vi "jacks_out_v3.vi"(0 "J4 DOWN":bool, 1 "J4 UP":bool, 2 "J3 DOWN":bool, 3 "J3 UP":bool, 4 "J2 DOWN":bool, 5 "J2 UP":bool, 6 "J1 DOWN":bool, 7 "J1 UP":bool) -> ()   [LabVIEW 2019]
uses:
  <vilib>/myRIO/Instrument Drivers/Onboard IO/UART/typedef/VISA Configuration.ctl
  <vilib>/Instr/_visa.llb/VISA Configure Serial Port (Instr).vi
  <vilib>/myRIO/Instrument Drivers/Onboard IO/UART/UART.lvlib
panel:
  out "resulting string":string
  out "Characters Read":string
  out "Character Count":u32
  in  "error in (no error)":errorcluster
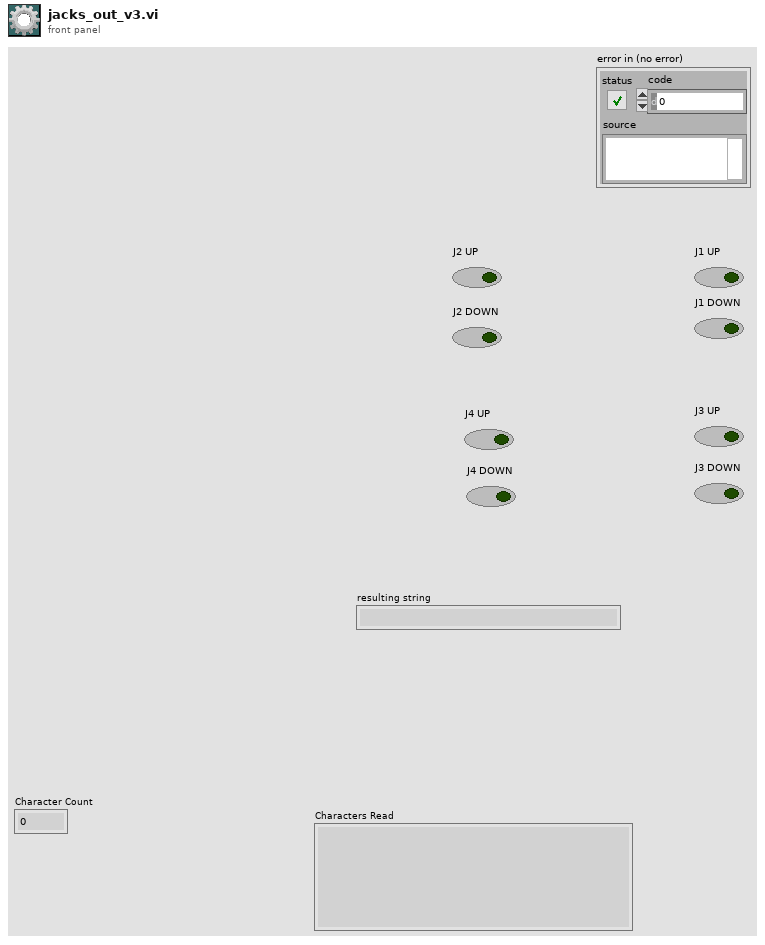
[diagram p1: front panel]
types:
  T1 = typedef "UART.lvlib/VISA Configuration.ctl" = cluster{"baud rate (9600)":u32, "data bits (8)":u16, "parity (0:none)":enum16{"None", "Odd", "Even", "Mark", "Space"}, "stop bits (10: 1 bit)":u16, "flow control (0:none)":u16, "termination char\n(0xA = '\\n' = LF) ":u8, "Enable Termination\nChar (T)":bool, "timeout (10sec)":u32}
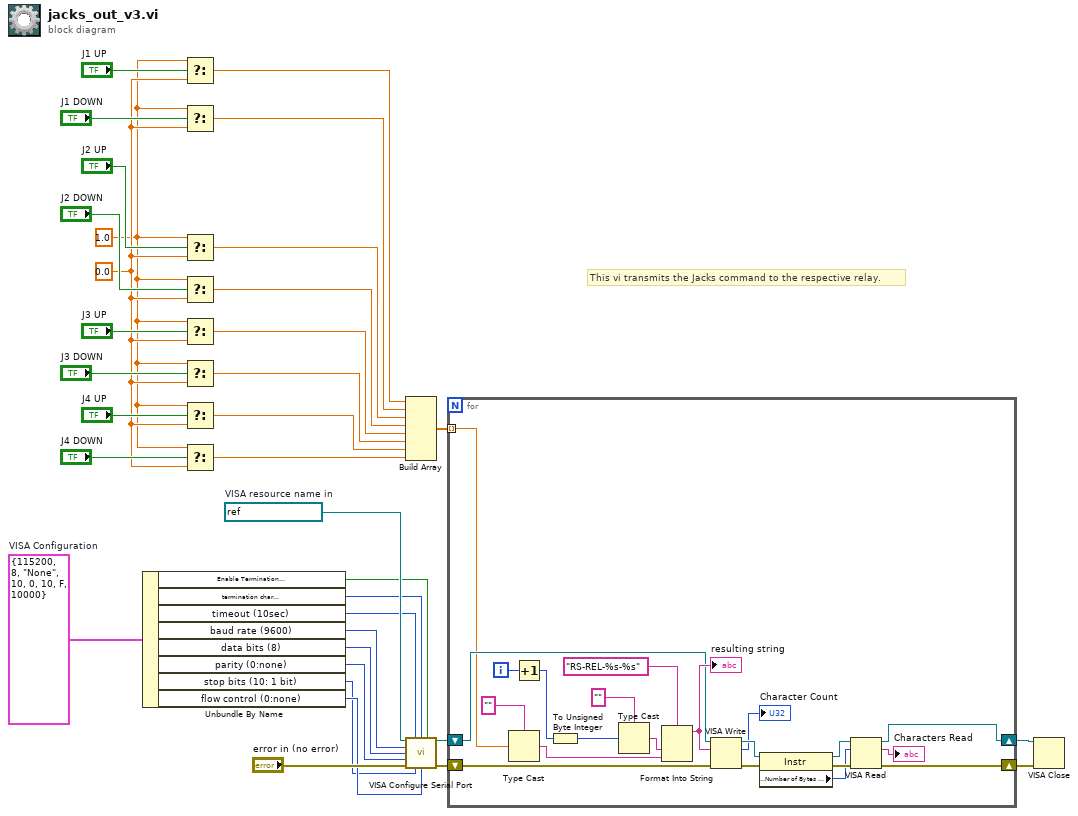
[diagram p0: block diagram]
diagram:
  w14 = 0.0 ("f")
  w13 = 1.0 ("t")
  w33 = T1 {"baud rate (9600)"=115200, "data bits (8)"=8, "parity (0:none)"=enum."None", "stop bits (10: 1 bit)"=10, "flow control (0:none)"=0, "termination char\n(0xA = '\\n' = LF) "=10, "Enable Termination\nChar (T)"=FALSE, "timeout (10sec)"=10000}  # VISA Configuration
  w34 = refnum<visa-resource-name> "ASRL2::INSTR"  # VISA resource name in
  # "This vi transmits the Jacks command to the respective relay."
  n1 = Unbundle By Name(w33) -> ("Enable Termination\nChar (T)"=w31:bool, "termination char\n(0xA = '\\n' = LF)"=w30:u8, "timeout (10sec)"=w29:u32, "baud rate (9600)"=w24:u32, "data bits (8)"=w25:u16, "parity (0:none)"=w26:enum16{"None", "Odd", "Even", "Mark", "Space"}, "stop bits (10: 1 bit)"=w27:u16, "flow control (0:none)"=w28:u16)
  n2 = Select(t=w13, s="J1 UP", f=w14) -> (s? t:f=w12:dbl)
  n3 = Select(t=w13, s="J1 DOWN", f=w14) -> (s? t:f=w11:dbl)
  n4 = Select(t=w13, s="J2 UP", f=w14) -> (s? t:f=w10:dbl)
  n5 = Select(t=w13, s="J2 DOWN", f=w14) -> (s? t:f=w9:dbl)
  n6 = Select(t=w13, s="J3 UP", f=w14) -> (s? t:f=w8:dbl)
  n7 = Select(t=w13, s="J3 DOWN", f=w14) -> (s? t:f=w7:dbl)
  n8 = Select(t=w13, s="J4 UP", f=w14) -> (s? t:f=w6:dbl)
  n9 = Select(t=w13, s="J4 DOWN", f=w14) -> (s? t:f=w5:dbl)
  n10 = Build Array(w12, w11, w10, w9, w8, w7, w6, w5) -> (w4:dbl[])
  n11 = call-poly "VISA Configure Serial Port"("VISA resource name"=w34, "timeout (10sec)"=w29, "termination char\n(0xA = '\\n' = LF)"=w30, "Enable Termination\nChar (T)"=w31, "baud rate (9600)"=w24, "data bits (8)"=w25, "parity (0:none)"=w26, "error in (no error)"="error in (no error)", "stop bits (10: 1 bit)"=w27, "flow control (0:none)"=w28) -> ("VISA resource name out"=w15:refnum<visa-resource-name>, "error out"=w1:errorcluster)  [unwired: 4 in]
  n12 = for {
    shift-right: [w37] -> w3
    shift-left: w15 -> [w41]
    tunnel: w4 -> [w39] mode=indexing
    shift-right: [w36] -> w2
    shift-left: w1 -> [w35]
    i -> [w40]
    n13 = Type Cast(type="", x=w39) -> (*(type *) &x=w52:string)
    n14 = Increment(x=w40) -> (x+1=w38:i32)
    n15 = To Unsigned Byte Integer(number=w38) -> (unsigned 8bit integer=w55:u8)
    n16 = Type Cast(type="", x=w55) -> (*(type *) &x=w53:string)
    n17 = Format Into String(format string="RS-REL-%s-%s", w53, w52) -> (resulting string=w54:string)  [unwired: 2 in, 1 out]
    "resulting string" <- w54
    n18 = VISA Write(VISA resource name=w41, write buffer=w54, error in (no error)=w35) -> (VISA resource name out=w49:refnum<visa-resource-name>, return count=→"Character Count":u32, error out=w50:errorcluster)
    n19 = property class="Instr"(reference=w49, error in=w50) -> (reference out=w48:refnum<visa-resource-name>, error out=w51:errorcluster, "Serial Settings:Number of Bytes at Serial Port"=w47:u32)
    n20 = VISA Read(VISA resource name=w48, byte count=w47, error in (no error)=w51) -> (VISA resource name out=w37:refnum<visa-resource-name>, read buffer=→"Characters Read":string, error out=w36:errorcluster)  [unwired: 1 out]
  }
  n21 = VISA Close(VISA resource name=w3, error in (no error)=w2) -> ()  [unwired: 1 out]
